vi "MTS_GenFileComment.vi"(7 "Measurement Type":T1(ring)=enum."Image File", 8 "error in":errorcluster, 9 "Upper Left":T3, 10 "Pixels":i32[](array[numeric]), 11 "Picture Size":dbl[](array[numeric])) -> (0 "error out":errorcluster, 2 "Image Info":T2, 3 "Comment":string)   [LabVIEW 8.6]
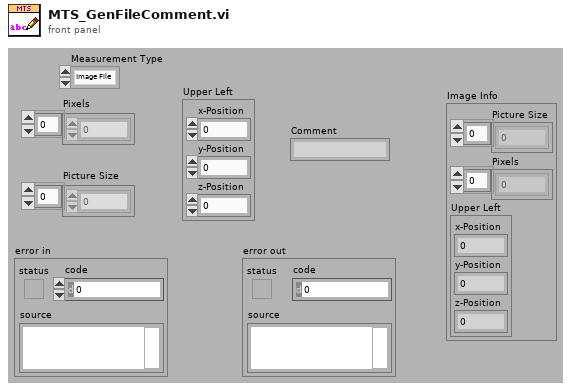
[diagram p1: front panel]
types:
  T1 = enum16{"not a pt3 File", "Image File", "Point Measurement", "Auto Point"}
  T2 = cluster{"Picture Size":dbl[], "Pixels":i32[], "Upper Left":cluster{"x-Position":dbl, "y-Position":dbl, "z-Position":dbl}}
  T3 = cluster{"x-Position":dbl, "y-Position":dbl, "z-Position":dbl}
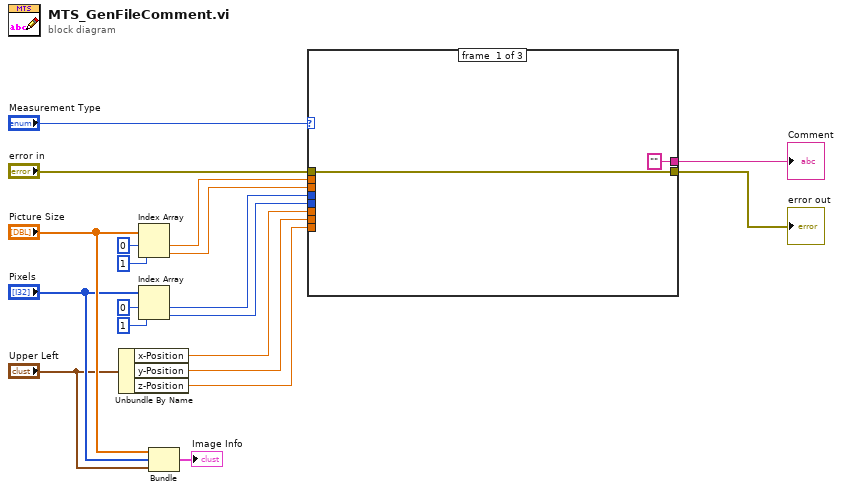
[diagram p0: block diagram]
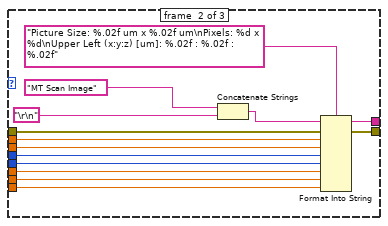
[diagram p2: hidden frame]
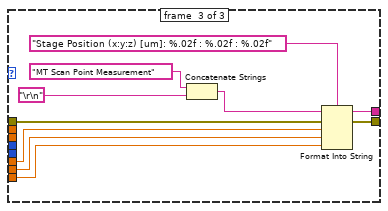
[diagram p3: hidden frame]
diagram:
  n1 = Unbundle By Name("Upper Left") -> ("x-Position"=w9:dbl, "y-Position"=w8:dbl, "z-Position"=w7:dbl)
  n2 = Index Array(array="Picture Size", index #1=0 ("index"), index #2=1 ("index")) -> (element #1=w13:dbl, element #2=w12:dbl)
  n3 = Index Array(array="Pixels", index #1=0 ("index"), index #2=1 ("index")) -> (element #1=w11:i32, element #2=w10:i32)
  n4 = Bundle("Picture Size"="Picture Size", "Pixels"="Pixels", "Upper Left"="Upper Left") -> (→"Image Info":T2)  [unwired: 1 in]
  n5 = case shown="\"Image File\"" "Measurement Type" {
    tunnel: [w21 w34 w44] -> w19
    tunnel: "error in" -> [w21 w33 w43]
    tunnel: w13 -> [_ w32 _]
    tunnel: w12 -> [_ w31 _]
    tunnel: w11 -> [_ w30 _]
    tunnel: w10 -> [_ w29 _]
    tunnel: w9 -> [_ w28 w41]
    tunnel: w8 -> [_ w27 w40]
    tunnel: w7 -> [_ w26 w39]
    tunnel: ["" w25 w42] -> w6
    frame #0 {
    }
    frame #1 {
      n6 = Concatenate Strings("MT Scan Image" ("initial string"), "\r\n") -> (w22:string)
      n7 = Format Into String(format string="Picture Size: %.02f um x %.02f um\nPixels: %d x %d\nUpper Left (x:y:z) [um]: %.02f : %.02f : %.02f", initial string=w22, error in=w33, w32, w31, w30, w29, w28, w27, w26) -> (resulting string=w25:string, error out=w34:errorcluster)
    }
    frame #2 {
      n8 = Concatenate Strings("MT Scan Point Measurement" ("initial string"), "\r\n") -> (w36:string)
      n9 = Format Into String(format string="Stage Position (x:y:z) [um]: %.02f : %.02f : %.02f", initial string=w36, error in=w43, w41, w40, w39) -> (resulting string=w42:string, error out=w44:errorcluster)
    }
  }
  "error out" <- w19
  "Comment" <- w6
